vi "niRFUtil MT UTIL Get Kaiser Filter Parameters.vi"(4 "ws":dbl=0.6, 6 "wp":dbl=0.4, 10 "len":i32=12, 11 "I":i32=128) -> (2 "Rs":dbl=8.0, 3 "beta":dbl)   [LabVIEW 2015, in "niRFUtil.lvlib"]
uses:
  niRFUtil.lvlib
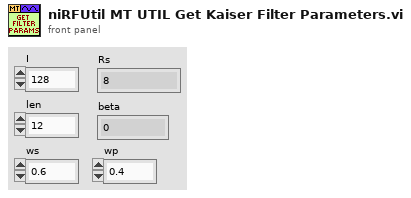
[diagram p1: front panel]
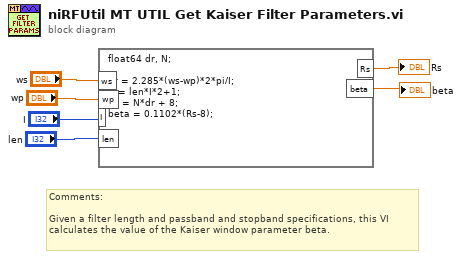
[diagram p0: block diagram]
diagram:
  # "Comments: \n\nGiven a filter length and passband and stopband specifications, this VI\ncalculates the value of the Kaiser window parameter beta."
  n1 = formula code="float64 dr, N;\n\ndr = 2.285*(ws-wp)*2*pi/I;\nN = len*I*2+1;\nRs = N*dr + 8;\nbeta = 0.1102*(Rs-8);"("ws"="ws", "wp"="wp", "I"="I", "len"="len") -> ("Rs"=→"Rs":dbl, "beta"=→"beta":dbl)
